vi "Measurement Parser.vi"(8 "error in (no error)":errorcluster, 9 "Universal Power Meter.lvlib:Universal Card.lvclass":refnum<class "Universal Card.lvclass">, 10 "Data Array":dbl[](array[numeric]), 11 "Tektronix PA1000 in":refnum<class "Tektronix PA1000.lvclass">) -> (0 "error out":errorcluster, 2 "Waveform Graph":dynamicdata(graph), 3 "Tektronix PA1000 out":refnum<class "Tektronix PA1000.lvclass">)   [LabVIEW 2013, in "Universal Power Meter.lvlib" / "Tektronix PA1000.lvlib" / "Tektronix PA1000.lvclass"]
uses:
  Tektronix PA1000.lvclass
  Universal Card Class/Universal Card.lvclass
  <instrlib>/Tektronix PA1000/Tektronix PA1000.lvlib
  Data Logger/Data Logger.lvclass
panel:
  out "Numeric":dbl
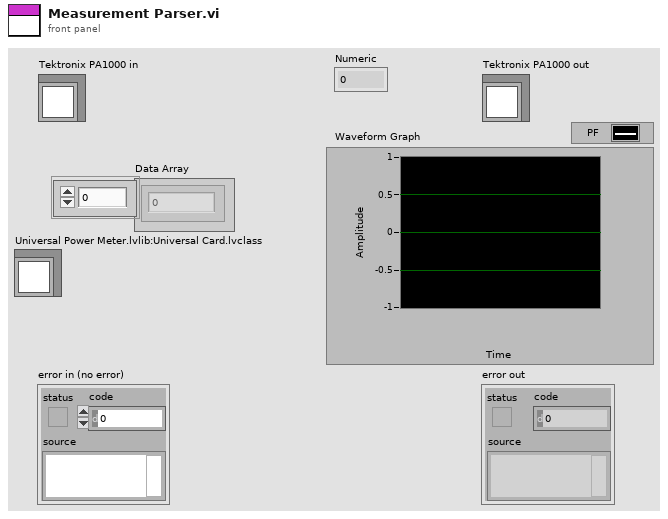
[diagram p1: front panel]
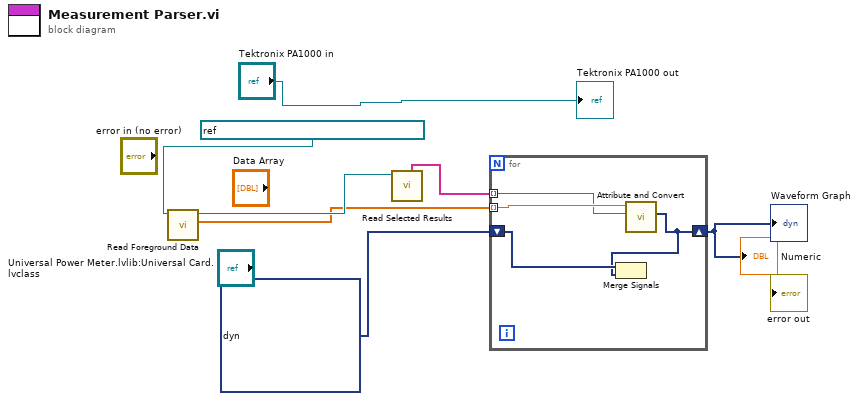
[diagram p0: block diagram]
diagram:
  n1 = call <instrlib>:"Read Foreground Data.vi"("VISA resource name"=refnum<visa-resource-name> "USB0::0x0699::0x4002::B010130::INSTR") -> ("Foreground Data"=w2:dbl[], "VISA resource name out"=w3:refnum<visa-resource-name>)  [unwired: 8 in, 1 out]
  n2 = call <instrlib>:"Read Selected Results.vi"("VISA resource name"=w3) -> ("Measurement List"=w7:string[])  [unwired: 6 in, 4 out]
  n3 = for {
    tunnel: w2 -> [w11] mode=indexing
    tunnel: w7 -> [w10] mode=indexing
    shift-right: [w8] -> w1
    shift-left: dynamicdata [] ("Waveform Graph 2") -> [w9]
    n4 = call "Attribute and Convert.vi"("Signal Name"=w10, "Number in"=w11) -> ("Dynamic Signal Out"=w8:dynamicdata)  [unwired: 9 in]
    n5 = Merge Signals(w9, w8) -> ()  [unwired: 1 out]
  }
  "Waveform Graph" <- w1
  "Numeric" <- w1
  "Tektronix PA1000 out" <- "Tektronix PA1000 in"
